vi "Read Col Header.vi"(7 "Section Name":string, 8 "error in (no error)":errorcluster, 11 "Config Data":T1(array[cluster])) -> (0 "error out":errorcluster, 1 "Data":string[][](array[string]), 2 "Column Header":string[](array[string]), 3 "Config Data dup":T1(array[cluster]), 4 "Section Find?":bool)   [LabVIEW 2020, in "GUCalibration2.lvlib"]
uses:
  GUCalibration2.lvlib
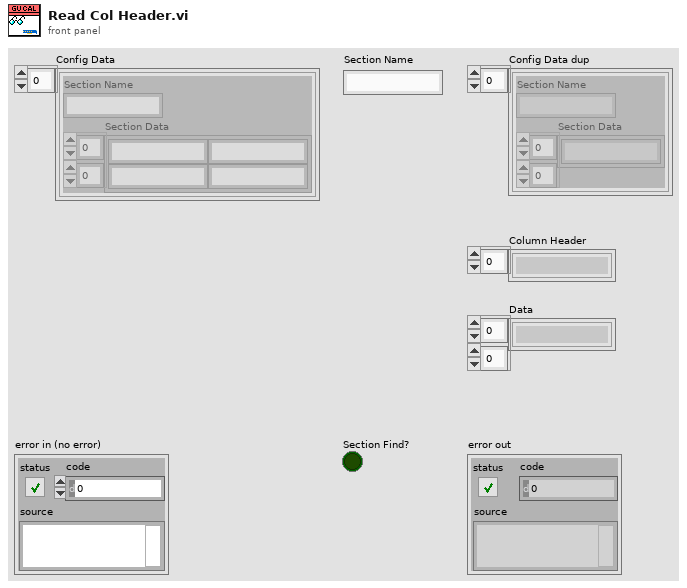
[diagram p1: front panel]
types:
  T1 = cluster{"Section Name":string, "Section Data":string[][]}[]
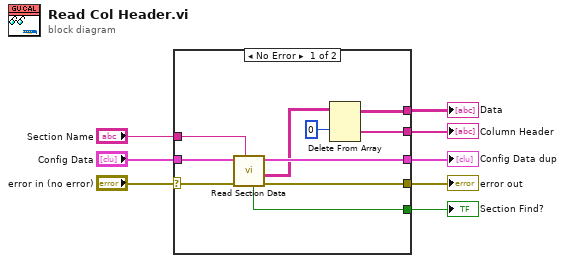
[diagram p0: block diagram]
diagram:
  n1 = case shown="No Error" "error in (no error)" {
    selector: "error in (no error)" -> [w16 w20]
    tunnel: "Section Name" -> [w17 _]
    tunnel: "Config Data" -> [w18 w19]
    tunnel: [w13 w20] -> w5
    tunnel: [w15 w19] -> w4
    tunnel: [w12 _] -> w3
    tunnel: [w11 _] -> w2
    tunnel: [w9 _] -> w1
    frame No Error {
      n2 = call "Read Section Data.vi"("Section Name"=w17, "error in (no error)"=w16, "Config Data"=w18) -> ("error out"=w13:errorcluster, "Section Data"=w14:string[][], "Config Data out"=w15:T1, "Section Exist"=w12:bool)  [unwired: 4 in, 1 out]
      n3 = Delete From Array(array=w14, index (row)=0 ("disabled index (col)")) -> (deleted portion=w11:string[], array with subset deleted=w9:string[][])  [unwired: 2 in]
    }
    frame Error {
    }
  }
  "error out" <- w5
  "Column Header" <- w2
  "Config Data dup" <- w4
  "Section Find?" <- w3
  "Data" <- w1
